vi "CSM - Check Status Registration.vi"(8 "error in (no error)":errorcluster, 10 "CSM Name":string, 11 "Broadcast state":string) -> (0 "error out":errorcluster, 3 "Array":T2(array[cluster]))   [LabVIEW 2020, in "Communicable State Machine.lvlib"]
uses:
  Communicable State Machine.lvlib
  CSM - Broadcast Message Type.ctl
  Trim Both Whitespace.vi
  global-CSMQ FGV Change Flag.vi
  global-Broadcast Cache Change Flag.vi
  Broadcast Item Key.vi
  _CSMOFGV.vi
  FGV-BroadcastRegistry.vi
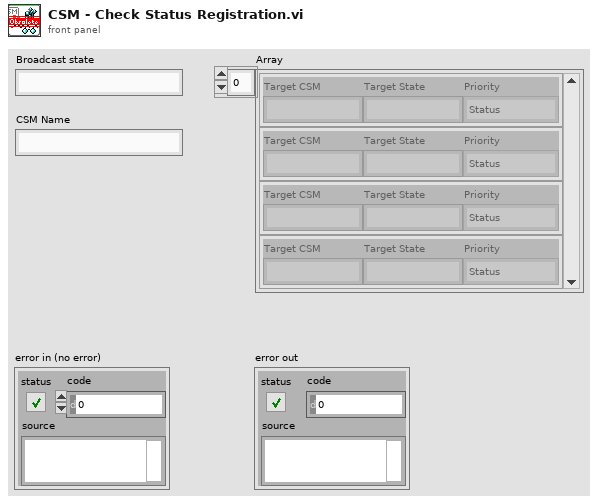
[diagram p1: front panel]
types:
  T1 = typedef "Communicable State Machine.lvlib/CSM - Broadcast Message Type.ctl" = enum16{"Status", "Interrupt(High)"}
  T2 = cluster{"Target CSM":string, "Target State":string, "Priority":T1}[]
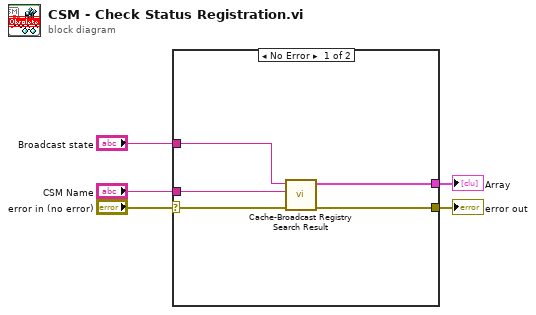
[diagram p0: block diagram]
diagram:
  n1 = case shown="No Error" "error in (no error)" {
    selector: "error in (no error)" -> [w7 w11]
    tunnel: "Broadcast state" -> [w10 _]
    tunnel: "CSM Name" -> [w9 _]
    tunnel: [w8 _] -> w3
    tunnel: [w6 w11] -> w1
    frame No Error {
      n2 = call "Cache-Broadcast Registry Search Result.vi"("error in (no error)"=w7, "CSM Name"=w9, "Broadcast state"=w10) -> ("error out"=w6:errorcluster, "Array"=w8:T2)  [unwired: 7 in]
    }
    frame Error {
    }
  }
  "Array" <- w3
  "error out" <- w1
